vi "CmdexPwmEnabled.vi"(8 "Uart Input":cluster{u64} {"?" format="%x"}, 9 "PWM Enabled":enum16{"DISABLED", "ENABLED", ""}(ring), 10 "PWM Id":enum16{"PWM0", "PWM1", "PWM2", "PWM3"}(ring), 11 "Error Input":errorcluster) -> (0 "Uart Output":cluster{u64} {"?" format="%x"}, 3 "Error Output":errorcluster)   [LabVIEW 2019]
doc: "<B>Cmdex</B>\nEnables or Disables the PWM."
uses:
  dll/LabViewUart.dll
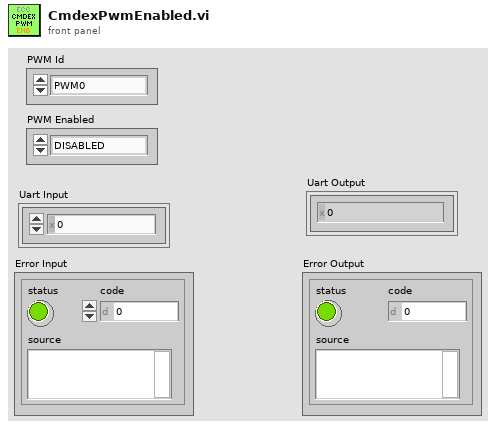
[diagram p1: front panel]
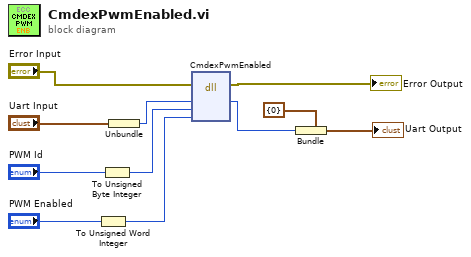
[diagram p0: block diagram]
diagram:
  n1 = To Unsigned Word Integer(number="PWM Enabled") -> (unsigned 16bit integer=w1:u16)
  n2 = To Unsigned Byte Integer(number="PWM Id") -> (unsigned 8bit integer=w6:u8)
  n3 = Unbundle("Uart Input") -> (w8:u64)
  n4 = dll-call lib="D:/Google Drive/INC-2020/INC352/INC352-2020/LabVIEW/examples/uart-cmdex/SubVI/dll/LabViewUart.dll" fn="CmdexPwmEnabled"(error in="Error Input", "Uart Handle"=w8, "id"=w6, "enabled"=w1) -> (error out=→"Error Output":errorcluster, "Uart Handle"=w3:u64)  [unwired: 5 in, 1 out]
  n5 = Bundle(cluster=cluster{u64} {0}, w3) -> (→"Uart Output":cluster{u64})
